vi "Send_command_and_check_response_string.vi"(3 "TimeOut Time (s)":dbl=30.0 format="%#_13g", 4 "milliseconds to wait":u32=5000, 5 "output cluster":T1 {"TimeStamp" format="%.2f"}, 6 "error in (no error)":errorcluster, 7 "Command":string="TIME", 8 "test response?":bool, 9 "Expected response":string) -> (0 "error IO":errorcluster, 1 "Return value":string)   [LabVIEW 2020]
uses:
  DataSocketCluster external.ctl
  vi Mode external.ctl
  04bf3837-9317-4129-9531-d6752085829f.vi
  <vilib>/Utility/error.llb/Error Cluster From Error Code.vi
  <vilib>/ErrorRing/Error Ring.xnode
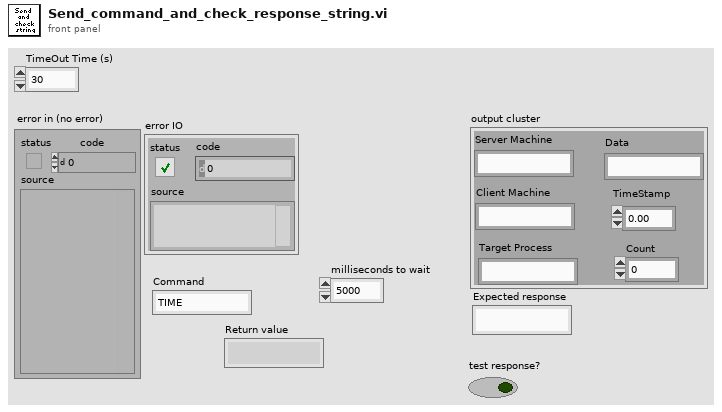
[diagram p1: front panel]
types:
  T1 = typedef "DataSocketCluster external.ctl" = cluster{"Server Machine":string, "Client Machine":string, "Data":string, "TimeStamp":dbl, "Count":i32, "Target Process":string}
  T2 = typedef "vi Mode external.ctl" = enum16{"Client", "Server"}
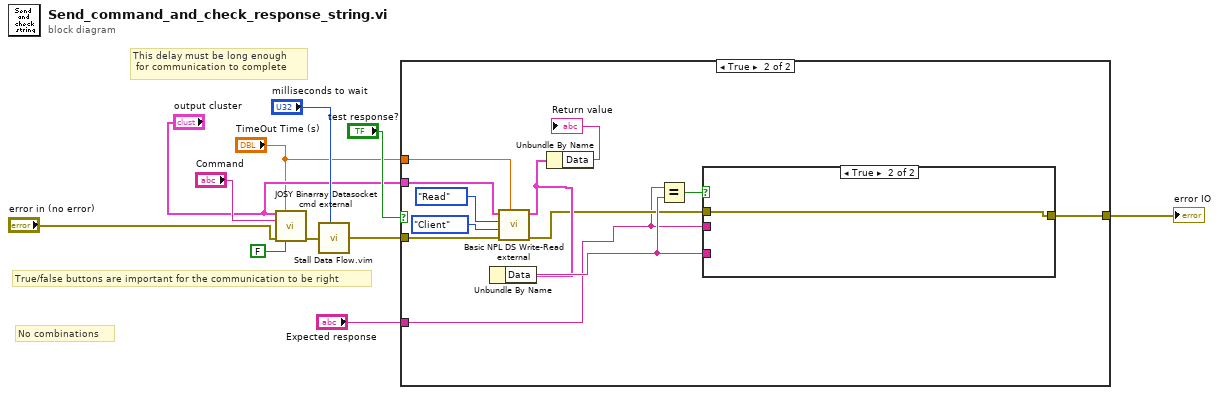
[diagram p0: block diagram]
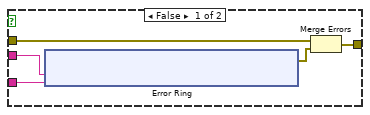
[diagram p3: hidden frame]
diagram:
  # "This delay must be long enough\n for communication to complete"
  # "No combinations"
  # "True/false buttons are important for the communication to be right"
  n1 = call "JOSY Binarray Datasocket cmd external.vi"("DataSocketCluster In"="output cluster", "TimeOut Time (s)"="TimeOut Time (s)", "Command"="Command", "error in (no error)"="error in (no error)", "Command has variable"=FALSE) -> ("error out"=w10:errorcluster)  [unwired: 7 in, 3 out]
  n2 = call "Stall Data Flow.vim"("value in"=w10, "milliseconds to wait"="milliseconds to wait") -> ("value out"=w9:errorcluster)  [unwired: 1 out]
  n3 = case shown="True" "test response?" {
    tunnel: w9 -> [w12 w24]
    tunnel: [w12 w19] -> w7
    tunnel: "Expected response" -> [_ w16]
    tunnel: "output cluster" -> [_ w15]
    tunnel: "TimeOut Time (s)" -> [_ w13]
    frame False {
    }
    frame True {
      n4 = call "Basic NPL DS Write-Read external.vi"("TimeOut Time (s)"=w13, "error in (no error)"=w24, "Server Mode"=vi_Mode_external."Client", "Operation Mode"=enum16{"Read", "Write", "Write/Read"}."Read", "DataSocketCluster In"=w15) -> ("error out"=w17:errorcluster, "DataSocketCluster Out"=w18:T1)  [unwired: 2 in, 1 out]
      n5 = Unbundle By Name(w18) -> ("Data"=w20:string)
      n6 = Unbundle By Name(w18) -> ("Data"=→"Return value":string)
      n7 = Equal?(x=w16, y=w20) -> (x = y?=w14:bool)
      n8 = case shown="True" w14 {
        tunnel: w17 -> [w26 w38]
        tunnel: w16 -> [w29 _]
        tunnel: w20 -> [w28 _]
        tunnel: [w25 w38] -> w19
        frame False {
          n9 = xnode "Error Ring"("parameter 0"=w29, "parameter 1"=w28) -> ("error out"=w27:errorcluster)
          n10 = Merge Errors(w26, w27) -> (w25:errorcluster)
        }
        frame True {
        }
      }
    }
  }
  "error IO" <- w7
